vi "DSF.Engine.Framework.Rx.End.vi"(8 "error in (no error)":errorcluster, 11 "Framework in":refnum<class "DSF.Engine.Framework.lvclass">) -> (0 "error out":errorcluster, 3 "Framework out":refnum<class "DSF.Engine.Framework.lvclass">)   [LabVIEW 2017, in "DSF.Engine.lvlib" / "DSF.Engine.Framework.lvclass"]
uses:
  DSF.Engine.Framework.lvclass
  DSF.Engine.Framework.lvclass/DSF.Engine.Framework.ctl
  Status/DSF.Engine.Status.Framework.lvclass/DSF.Engine.Status.Framework.ctl
  Status/DSF.Engine.Status.Framework.Performance.lvclass/DSF.Engine.Status.Framework.Performance.ctl
  <vilib>/National Instruments/Memory Manager/Classes/Pointer/Memory.Pointer.lvclass/Memory.Pointer.ctl
  <vilib>/National Instruments/Memory Manager/Classes/Pointer/Memory.Pointer.Write.vi
  <vilib>/National Instruments/Memory Manager/Classes/Pointer/Memory.Pointer.Write.0D.U32.vi
  <vilib>/National Instruments/Memory Manager/Classes/Pointer/Memory.Pointer.Write.No Check.0D.U32.vi
  <vilib>/National Instruments/Memory Manager/Classes/Pointer/Memory.Pointer.Parameter Check.Null Pointer.vi
  <vilib>/National Instruments/Memory Manager/Classes/Pointer/Memory.Pointer.Parameter Check.Subset.vi
  <vilib>/National Instruments/Memory Manager/Classes/Pointer/Memory.Pointer.Get Address.vi
  <vilib>/National Instruments/Memory Manager/Classes/Pointer/Memory.Pointer.Errors.vi
  <vilib>/National Instruments/Memory Manager/Classes/Pointer/Memory.Pointer.Errors.Null Pointer.vi
  <vilib>/National Instruments/Memory Manager/Classes/Pointer/Memory.Pointer.Errors.Out of Bounds.vi
  <vilib>/National Instruments/Memory Manager/Classes/Pointer/Memory.Pointer.Get Size.vi
  <vilib>/National Instruments/Memory Manager/Classes/Pointer/Memory.Pointer.Errors.Create Error.vi
  <vilib>/NI/Static Error Handling/VIs/Static Error Handling.Source Buffer.Write.String.vi
  <vilib>/National Instruments/Memory Manager/Classes/Pointer/Memory.Pointer.Errors.Write Pointer Size.vi
  <vilib>/NI/Static Error Handling/VIs/Static Error Handling.Source Buffer.Write.Numeric.Scalar.Base10.vi
  <vilib>/NI/Static Error Handling/VIs/Static Error Handling.Source Buffer.Write.Numeric.Scalar.Base10 (U64).vi
  <vilib>/NI/Static Error Handling/VIs/Static Error Handling.Error Cluster Constant.vi
  <vilib>/NI/Static Error Handling/VIs/Static Error Handling.Error Cluster Constant (512B).vi
  <vilib>/NI/Static Error Handling/VIs/Static Error Handling.Parameters.Status.Set.vi
  <vilib>/NI/Static Error Handling/VIs/Static Error Handling.Parameters.Code.Set.vi
  <vilib>/NI/Static Error Handling/VIs/Static Error Handling.Parameters.VI Source.Set.vi
  <vilib>/National Instruments/Memory Manager/Constants/Memory.Constants.vi
  <vilib>/National Instruments/Memory Manager/Constants/Memory.Constants.Library Name.vi
  <vilib>/National Instruments/Memory Manager/Classes/Pointer/Memory.Pointer.Errors.Get Info.vi
  Status/DSF.Engine.Status.Framework.lvclass
  Status/DSF.Engine.Status.Framework.Performance.lvclass
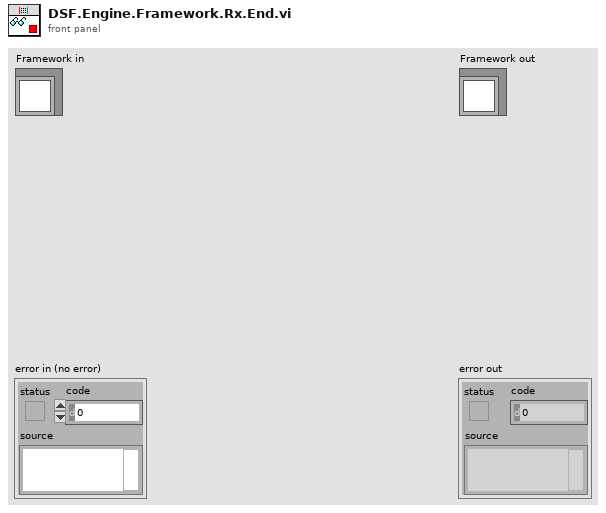
[diagram p1: front panel]
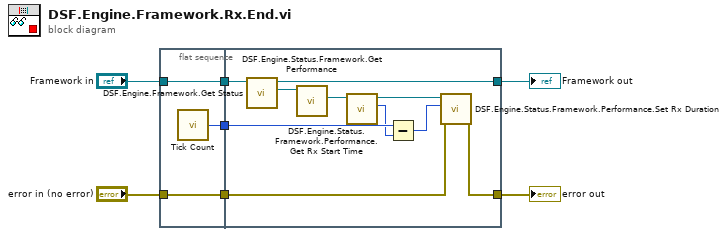
[diagram p0: block diagram]
diagram:
  n1 = flat-sequence {
    tunnel: "Framework in" -> [w10]
    tunnel: [w10] -> w5
    tunnel: [w9] -> w4
    tunnel: "error in (no error)" -> [w8]
    tunnel: [w8] -> w2
    tunnel: [w18] -> w6
    tunnel: w5 -> [w19]
    tunnel: w4 -> [w16]
    tunnel: w2 -> [w12]
    tunnel: [w11] -> w1
    frame #0 {
      n2 = call "Tick Count"() -> ("Tick Count(uSec)"=w9:u32)
    }
    frame #1 {
      n3 = call "DSF.Engine.Framework.Get Status.vi"("Framework in"=w19) -> ("Status"=w20:refnum<class "DSF.Engine.Status.Framework.lvclass">, "Framework out"=w18:refnum<class "DSF.Engine.Framework.lvclass">)  [unwired: 9 in]
      n4 = call "DSF.Engine.Status.Framework.Get Performance.vi"("Framework Status in"=w20) -> ("Framework Performance"=w17:refnum<class "DSF.Engine.Status.Framework.Performance.lvclass">)  [unwired: 9 in, 1 out]
      n5 = call "DSF.Engine.Status.Framework.Performance.Get Rx Start Time.vi"("Framework Performance in"=w17) -> ("Rx start time"=w15:u32, "Framework Performance out"=w14:refnum<class "DSF.Engine.Status.Framework.Performance.lvclass">)  [unwired: 9 in]
      n6 = Subtract(x=w16, y=w15) -> (x-y=w13:u32)
      n7 = call "DSF.Engine.Status.Framework.Performance.Set Rx Duration.vi"("error in (no error)"=w12, "rx duration"=w13, "Framework Performance in"=w14) -> ("error out"=w11:errorcluster)  [unwired: 7 in, 1 out]
    }
  }
  "error out" <- w1
  "Framework out" <- w6
